vi "SUMMER SUNDAY BYTE[2].vi"() -> ()   [LabVIEW 2009]
uses:
  <vilib>/ULx/Create Channel.llb/ULx Create Channel (AI-Voltage-Basic).vi
  <vilib>/ULx/Read.llb/ULx Read (Analog DBL 1Chan 1Samp).vi
panel:
  out "POWER":bool
  out "data":dbl format="%_6g"
  out "xray":bool caption="BitValue"
  out "ENERGY LEVEL":dbl(knob) scale=0.0..15.0
  out "x*y":dbl
  out "Beam Pot":dbl format="%_6g"
  out "READY 2":bool
  out "DUMP":bool
  out "POWER":bool
  out "?":bool
  out "?":bool
  out "?":bool
  out "?":bool
  out "?":bool
  out "?":bool
  out "?":bool
  out "?":bool
  out "?":bool
  out "?":bool
  out "OPEN":bool
  out "CLOSED":bool
  out "READY":bool
  out "FAULT":bool
  out "MAGNET FORCE":dbl(slide) scale=0.0..10.0
  out "READY":bool
  out "TEMPERATURE":dbl(slide) scale=0.0..100.0
  in  "stop":bool
  out "?":bool
  out "?":bool
  out "?":bool
  out "?":bool
  out "FAULT":bool
  out "POWER":bool
  out "FLOW IN GPM":dbl(knob) scale=0.0..15.0
  # "USERS LAB AREA"
  # "BEAM STATUS"
  # "ROOM"
  # "XRAY"
  # "PUMP STATION"
  # "MAGNET STATUS"
  # "ORBIT"
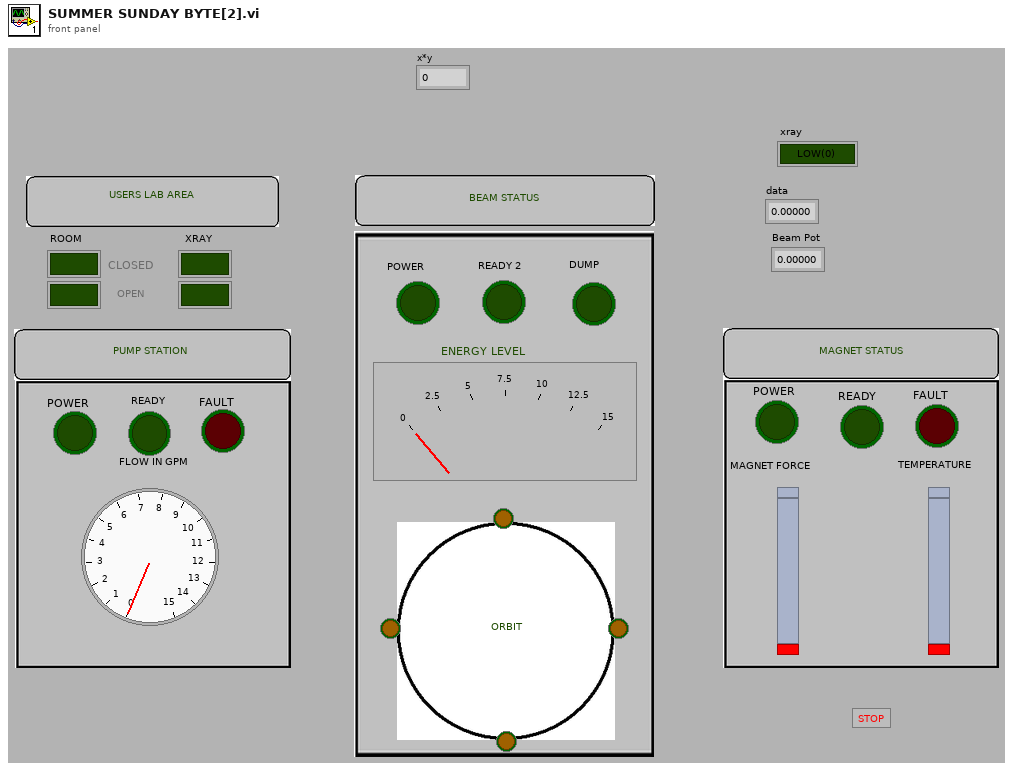
[diagram p1: front panel]
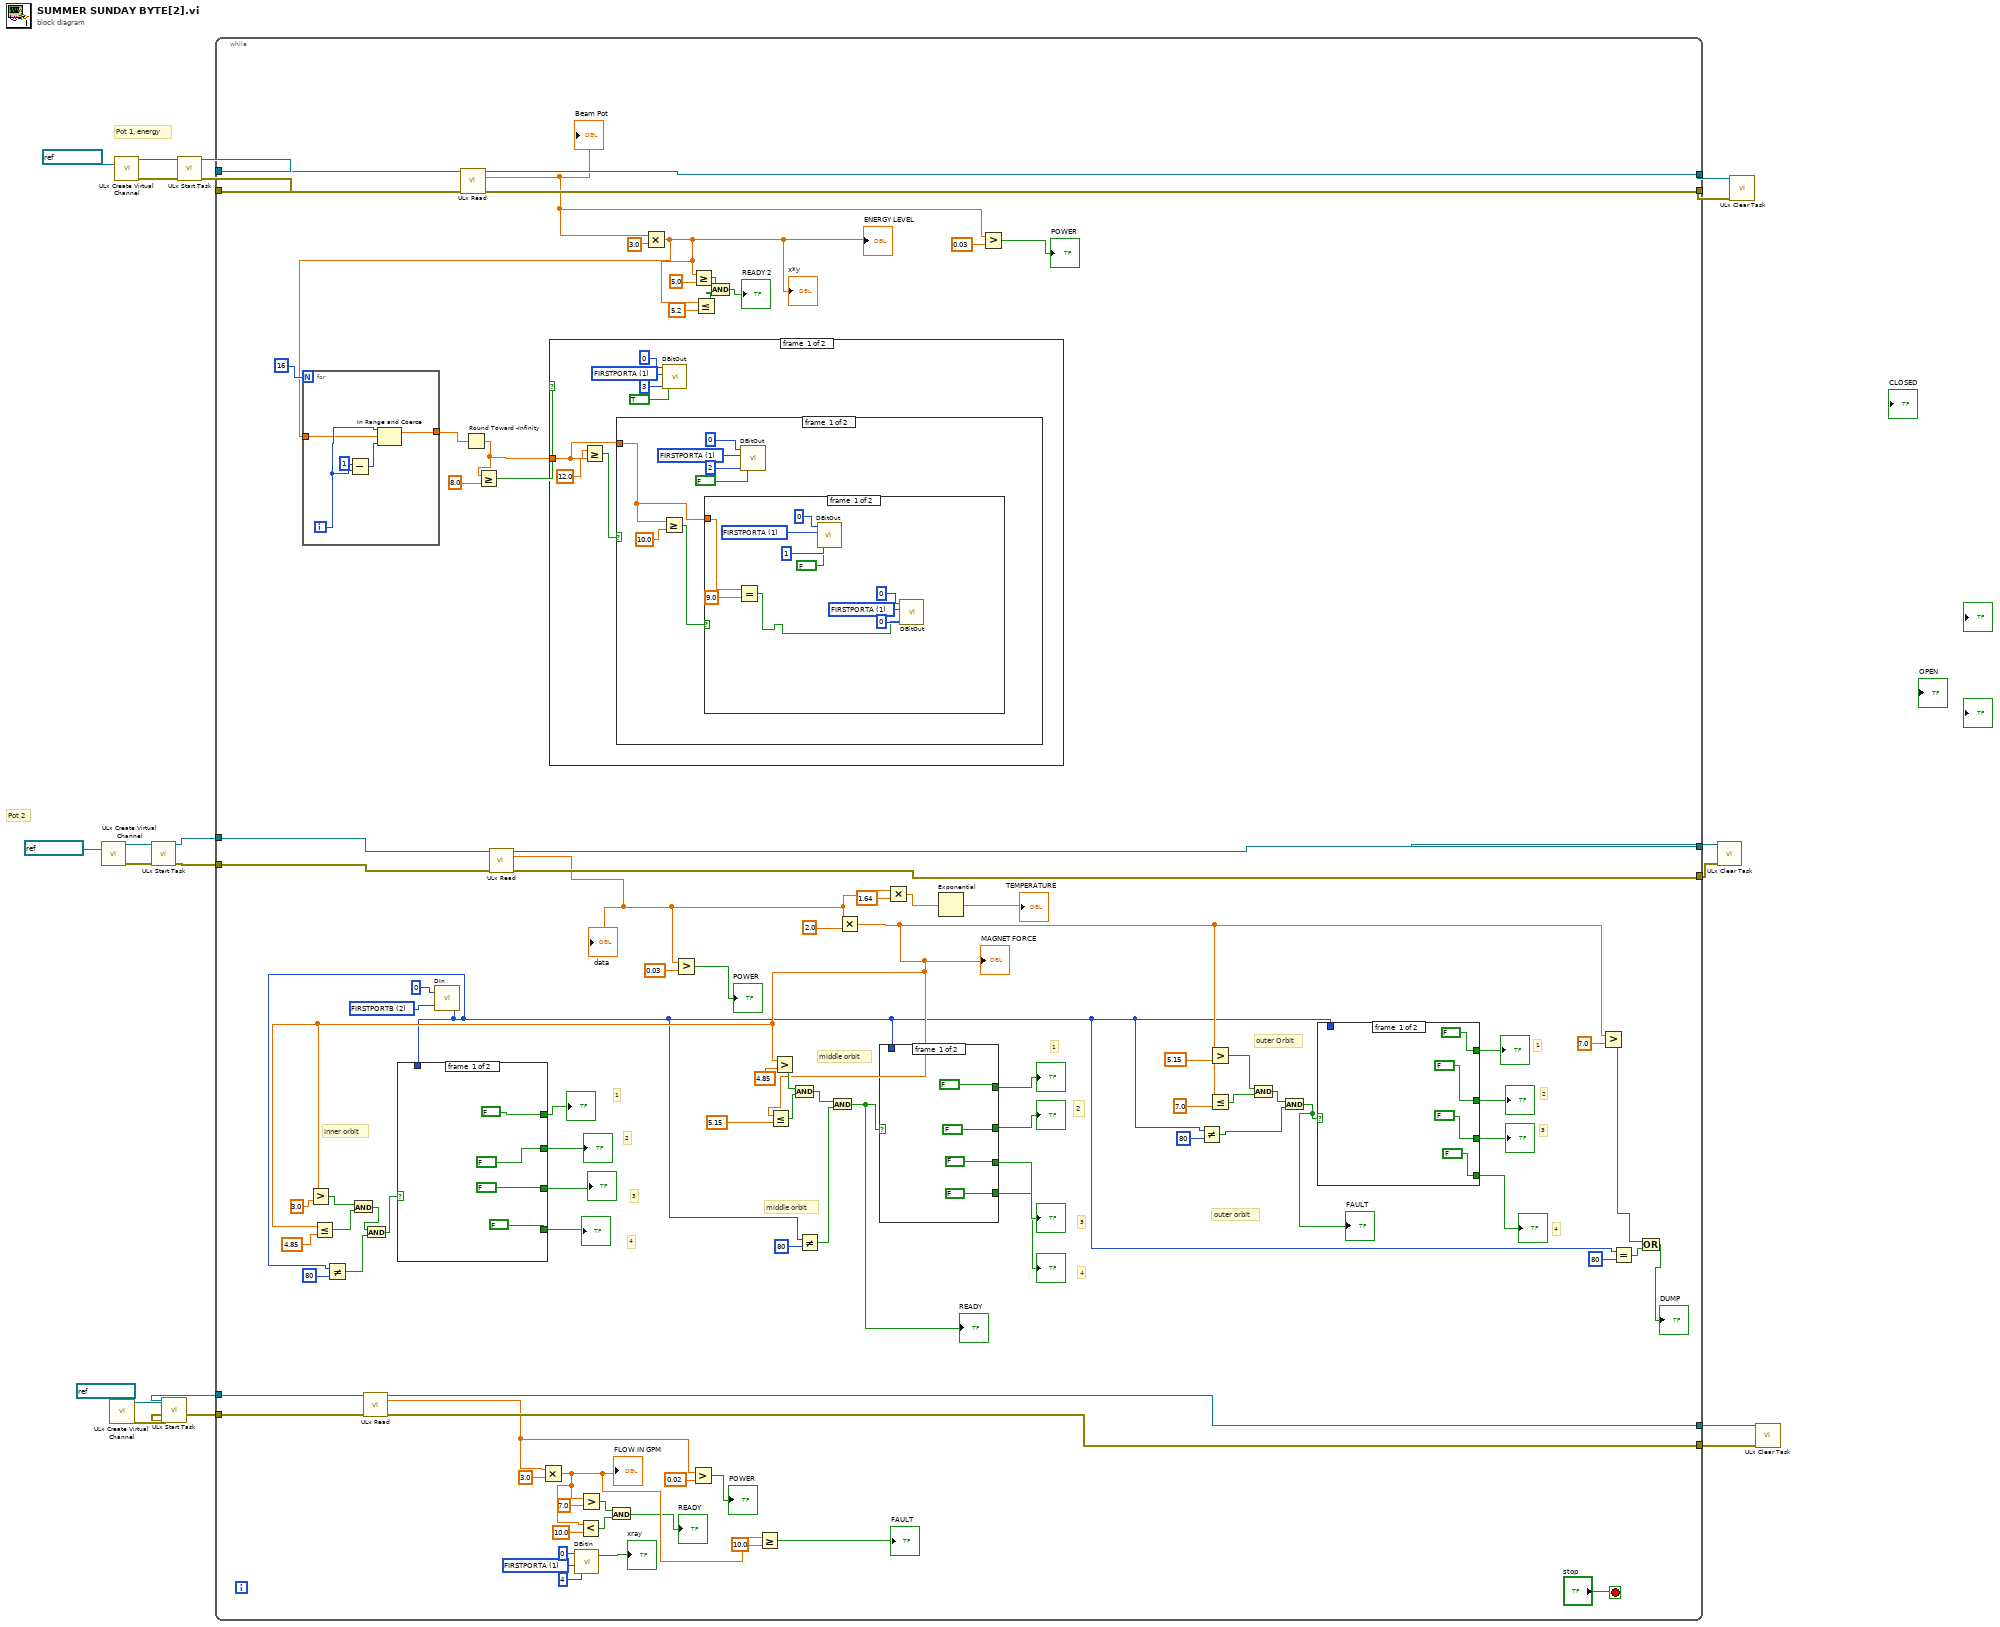
[diagram p0: block diagram]
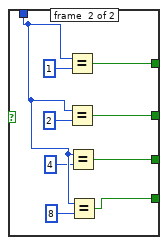
[diagram p2: hidden frame]
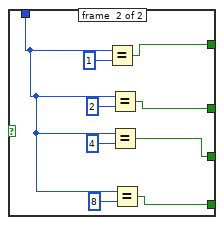
[diagram p3: hidden frame]
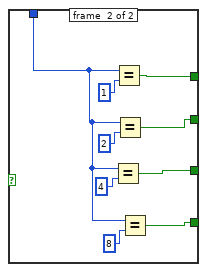
[diagram p4: hidden frame]
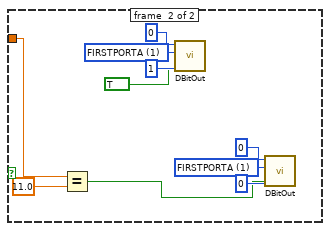
[diagram p5: hidden frame]
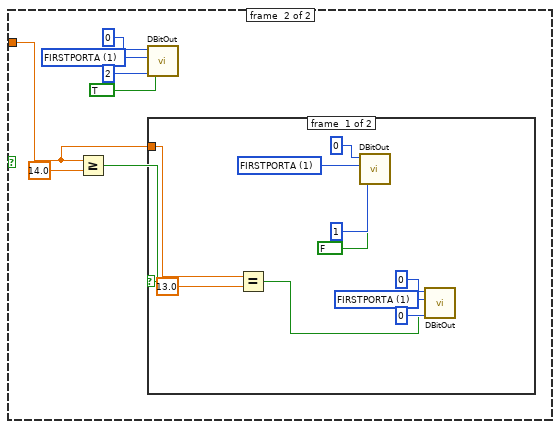
[diagram p6: hidden frame]
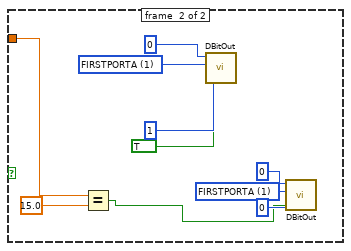
[diagram p7: hidden frame]
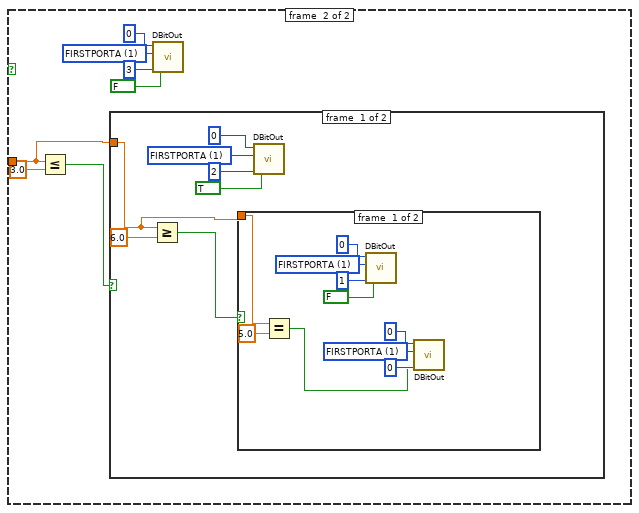
[diagram p8: hidden frame]
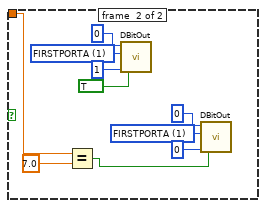
[diagram p9: hidden frame]
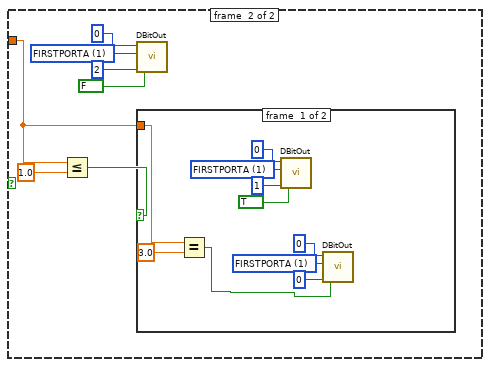
[diagram p10: hidden frame]
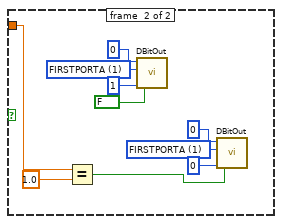
[diagram p11: hidden frame]
diagram:
  # "Pot 2"
  # "Pot 1, energy"
  n1 = call-poly <vilib>:"ULx Create Virtual Channel.vi"("physical channels"=refnum<k21> "Dev0/Ai1") -> ("task out"=w15:refnum<k24>, "error out"=w14:errorcluster)  [unwired: 13 in]
  n2 = call-poly <vilib>:"ULx Create Virtual Channel.vi"("physical channels"=refnum<k21> "Dev0/Ai2") -> ("task out"=w7:refnum<k24>, "error out"=w6:errorcluster)  [unwired: 13 in]
  n3 = call-poly <vilib>:"ULx Create Virtual Channel.vi"("physical channels"=refnum<k21> "Dev0/Ai0") -> ("task out"=w21:refnum<k24>, "error out"=w20:errorcluster)  [unwired: 13 in]
  n4 = call <vilib>:"ULx Start Task.vi"("task in"=w15, "error in"=w14) -> ("task out"=w13:refnum<k24>, "error out"=w12:errorcluster)  [unwired: 12 in]
  n5 = call <vilib>:"ULx Start Task.vi"("task in"=w7, "error in"=w6) -> ("task out"=w5:refnum<k24>, "error out"=w4:errorcluster)  [unwired: 12 in]
  n6 = call <vilib>:"ULx Start Task.vi"("task in"=w21, "error in"=w20) -> ("task out"=w19:refnum<k24>, "error out"=w18:errorcluster)  [unwired: 12 in]
  n7 = while {
    tunnel: w19 -> [w116]
    tunnel: w18 -> [w115]
    tunnel: [w114] -> w17
    tunnel: [w113] -> w16
    tunnel: w13 -> [w106]
    tunnel: w12 -> [w105]
    tunnel: [w104] -> w11
    tunnel: [w103] -> w10
    tunnel: w5 -> [w61]
    tunnel: w4 -> [w60]
    tunnel: [w59] -> w2
    tunnel: [w58] -> w1
    stop <- "stop" stop-if-true
    w56 = 1 items=["AUXPORT", "FIRSTPORTA"] ("PortType")
    w80 = 2 items=["AUXPORT", "FIRSTPORTA", "FIRSTPORTB", "FIRSTPORTCL", "FIRSTPORTCH", "SECONDPORTA", "SECONDPORTB", "SECONDPORTCL", "SECONDPORTCH", "THIRDPORTA", "THIRDPORTB", "THIRDPORTCL", "THIRDPORTCH", "FOURTHPORTA", "FOURTHPORTB", "FOURTHPORTCL", "FOURTHPORTCH", "FIFTHPORTA", "FIFTHPORTB", "FIFTHPORTCL", "FIFTHPORTCH", "SIXTHPORTA", "SIXTHPORTB", "SIXTHPORTCL", "SIXTHPORTCH", "SEVENTHPORTA", "SEVENTHPORTB", "SEVENTHPORTCL", "SEVENTHPORTCH", "EIGTHPORTA", "EIGHTHPORTB", "EIGHTHPORTCL", "EIGHTHPORTCH"] ("PortNum")
    # "outer Orbit"
    # "middle orbit"
    # "4"
    # "3"
    # "2"
    # "1"
    # "1"
    # "2"
    # "3"
    # "4"
    # "4"
    # "3"
    # "2"
    # "1"
    # "outer orbit"
    # "inner orbit"
    # "middle orbit"
    n8 = call-poly <vilib>:"ULx Read.vi"("task in"=w61, "error in"=w60) -> ("task out"=w59:refnum<k24>, "data"=w47:dbl, "error out"=w58:errorcluster)  [unwired: 11 in]
    n9 = call <menus>:"DIn.VI"("PortNum"=w80, "BoardNum"=u32 0) -> ("DataValue"=w68:i16)  [unwired: 1 out]
    n10 = Not Equal?(x=w68, y=i16 80) -> (x != y?=w90:bool)
    n11 = call-poly <vilib>:"ULx Read.vi"("task in"=w116, "error in"=w115) -> ("task out"=w114:refnum<k24>, "data"=w49:dbl, "error out"=w113:errorcluster)  [unwired: 11 in]
    "Beam Pot" <- w49
    n12 = call-poly <vilib>:"ULx Read.vi"("task in"=w106, "error in"=w105) -> ("task out"=w104:refnum<k24>, "data"=w25:dbl, "error out"=w103:errorcluster)  [unwired: 11 in]
    "data" <- w25
    n13 = Multiply(x=w47, y=3.0) -> (x*y=w32:dbl)
    "FLOW IN GPM" <- w32
    n14 = call <menus>:"DBitIn.VI"("BitNum"=4, "PortType"=w56, "BoardNum"=u32 0) -> ("BitValue"=→"xray":bool)  [unwired: 1 out]
    n15 = Less?(x=w32, y=10.0) -> (x < y?=w30:bool)
    n16 = Greater?(x=w32, y=7.0) -> (0:w31:bool)
    n17 = And(x=w31, y=w30) -> (x .and. y?=→"READY":bool)
    n18 = Multiply(x=w49, y=3.0) -> (x*y=w42:dbl)
    "x*y" <- w42
    "ENERGY LEVEL" <- w42
    n19 = for {
      N: 16 -> [_]
      tunnel: w42 -> [w280]
      tunnel: [w279] -> w110
      i -> [w282]
      n20 = Subtract(x=1, y=w282) -> (x-y=w283:i32)
      n21 = In Range and Coerce(upper limit=w282, x=w280, lower limit=w283) -> (coerced(x)=w279:dbl)  [unwired: 1 out]
    }
    n22 = Round Toward -Infinity(1:w110) -> (0:w107:dbl)
    n23 = Greater Or Equal?(x=w107, y=8.0) -> (x >= y?=w108:bool)
    n24 = case shown="False" w108 {
      tunnel: w107 -> [w157 w218]
      frame #0 {
        w162 = u32 1 items=["AUXPORT", "FIRSTPORTA"] ("PortType")
        n25 = Greater Or Equal?(x=w157, y=12.0) -> (x >= y?=w158:bool)
        n26 = case shown="True" w158 {
          tunnel: w157 -> [w164 w191]
          frame #0 {
            w169 = u32 1 items=["AUXPORT", "FIRSTPORTA"] ("PortType")
            n27 = Greater Or Equal?(x=w164, y=10.0) -> (x >= y?=w165:bool)
            n28 = case shown="True" w165 {
              tunnel: w164 -> [w176 w187]
              frame #0 {
                w174 = u32 1 items=["AUXPORT", "FIRSTPORTA"] ("PortType")
                w179 = u32 1 items=["AUXPORT", "FIRSTPORTA"] ("PortType")
                n29 = Equal?(x=w176, y=9.0) -> (x = y?=w171:bool)
                n30 = call <menus>:"DBitOut.VI"("BitValue"=FALSE, "BitNum"=u32 1, "PortType"=w179, "BoardNum"=u32 0) -> ()  [unwired: 1 out]
                n31 = call <menus>:"DBitOut.VI"("BitValue"=w171, "BitNum"=u32 0, "PortType"=w174, "BoardNum"=u32 0) -> ()  [unwired: 1 out]
              }
              frame #1 {
                w184 = u32 1 items=["AUXPORT", "FIRSTPORTA"] ("PortType")
                w189 = u32 1 items=["AUXPORT", "FIRSTPORTA"] ("PortType")
                n32 = Equal?(x=w187, y=11.0) -> (x = y?=w181:bool)
                n33 = call <menus>:"DBitOut.VI"("BitValue"=TRUE, "BitNum"=u32 1, "PortType"=w189, "BoardNum"=u32 0) -> ()  [unwired: 1 out]
                n34 = call <menus>:"DBitOut.VI"("BitValue"=w181, "BitNum"=u32 0, "PortType"=w184, "BoardNum"=u32 0) -> ()  [unwired: 1 out]
              }
            }
            n35 = call <menus>:"DBitOut.VI"("BitValue"=FALSE, "BitNum"=u32 2, "PortType"=w169, "BoardNum"=u32 0) -> ()  [unwired: 1 out]
          }
          frame #1 {
            w196 = u32 1 items=["AUXPORT", "FIRSTPORTA"] ("PortType")
            n36 = Greater Or Equal?(x=w191, y=14.0) -> (x >= y?=w192:bool)
            n37 = call <menus>:"DBitOut.VI"("BitValue"=TRUE, "BitNum"=u32 2, "PortType"=w196, "BoardNum"=u32 0) -> ()  [unwired: 1 out]
            n38 = case shown="False" w192 {
              tunnel: w191 -> [w203 w213]
              frame #0 {
                w201 = u32 1 items=["AUXPORT", "FIRSTPORTA"] ("PortType")
                w206 = u32 1 items=["AUXPORT", "FIRSTPORTA"] ("PortType")
                n39 = Equal?(x=w203, y=13.0) -> (x = y?=w198:bool)
                n40 = call <menus>:"DBitOut.VI"("BitValue"=FALSE, "BitNum"=u32 1, "PortType"=w206, "BoardNum"=u32 0) -> ()  [unwired: 1 out]
                n41 = call <menus>:"DBitOut.VI"("BitValue"=w198, "BitNum"=u32 0, "PortType"=w201, "BoardNum"=u32 0) -> ()  [unwired: 1 out]
              }
              frame #1 {
                w211 = u32 1 items=["AUXPORT", "FIRSTPORTA"] ("PortType")
                w216 = u32 1 items=["AUXPORT", "FIRSTPORTA"] ("PortType")
                n42 = Equal?(x=w213, y=15.0) -> (x = y?=w208:bool)
                n43 = call <menus>:"DBitOut.VI"("BitValue"=TRUE, "BitNum"=u32 1, "PortType"=w216, "BoardNum"=u32 0) -> ()  [unwired: 1 out]
                n44 = call <menus>:"DBitOut.VI"("BitValue"=w208, "BitNum"=u32 0, "PortType"=w211, "BoardNum"=u32 0) -> ()  [unwired: 1 out]
              }
            }
          }
        }
        n45 = call <menus>:"DBitOut.VI"("BitValue"=TRUE, "BitNum"=u32 3, "PortType"=w162, "BoardNum"=u32 0) -> ()  [unwired: 1 out]
      }
      frame #1 {
        w223 = u32 1 items=["AUXPORT", "FIRSTPORTA"] ("PortType")
        n46 = Less Or Equal?(x=w218, y=3.0) -> (x <= y?=w219:bool)
        n47 = case shown="False" w219 {
          tunnel: w218 -> [w225 w252]
          frame #0 {
            w230 = u32 1 items=["AUXPORT", "FIRSTPORTA"] ("PortType")
            n48 = Greater Or Equal?(x=w225, y=6.0) -> (x >= y?=w226:bool)
            n49 = case shown="False" w226 {
              tunnel: w225 -> [w234 w247]
              frame #0 {
                w236 = u32 1 items=["AUXPORT", "FIRSTPORTA"] ("PortType")
                w240 = u32 1 items=["AUXPORT", "FIRSTPORTA"] ("PortType")
                n50 = Equal?(x=w234, y=5.0) -> (x = y?=w232:bool)
                n51 = call <menus>:"DBitOut.VI"("BitValue"=FALSE, "BitNum"=u32 1, "PortType"=w240, "BoardNum"=u32 0) -> ()  [unwired: 1 out]
                n52 = call <menus>:"DBitOut.VI"("BitValue"=w232, "BitNum"=u32 0, "PortType"=w236, "BoardNum"=u32 0) -> ()  [unwired: 1 out]
              }
              frame #1 {
                w244 = u32 1 items=["AUXPORT", "FIRSTPORTA"] ("PortType")
                w250 = u32 1 items=["AUXPORT", "FIRSTPORTA"] ("PortType")
                n53 = Equal?(x=w247, y=7.0) -> (x = y?=w242:bool)
                n54 = call <menus>:"DBitOut.VI"("BitValue"=TRUE, "BitNum"=u32 1, "PortType"=w250, "BoardNum"=u32 0) -> ()  [unwired: 1 out]
                n55 = call <menus>:"DBitOut.VI"("BitValue"=w242, "BitNum"=u32 0, "PortType"=w244, "BoardNum"=u32 0) -> ()  [unwired: 1 out]
              }
            }
            n56 = call <menus>:"DBitOut.VI"("BitValue"=TRUE, "BitNum"=u32 2, "PortType"=w230, "BoardNum"=u32 0) -> ()  [unwired: 1 out]
          }
          frame #1 {
            w257 = u32 1 items=["AUXPORT", "FIRSTPORTA"] ("PortType")
            n57 = Less Or Equal?(x=w252, y=1.0) -> (x <= y?=w253:bool)
            n58 = call <menus>:"DBitOut.VI"("BitValue"=FALSE, "BitNum"=u32 2, "PortType"=w257, "BoardNum"=u32 0) -> ()  [unwired: 1 out]
            n59 = case shown="True" w253 {
              tunnel: w252 -> [w264 w274]
              frame #0 {
                w261 = u32 1 items=["AUXPORT", "FIRSTPORTA"] ("PortType")
                w267 = u32 1 items=["AUXPORT", "FIRSTPORTA"] ("PortType")
                n60 = Equal?(x=w264, y=3.0) -> (x = y?=w259:bool)
                n61 = call <menus>:"DBitOut.VI"("BitValue"=TRUE, "BitNum"=u32 1, "PortType"=w267, "BoardNum"=u32 0) -> ()  [unwired: 1 out]
                n62 = call <menus>:"DBitOut.VI"("BitValue"=w259, "BitNum"=u32 0, "PortType"=w261, "BoardNum"=u32 0) -> ()  [unwired: 1 out]
              }
              frame #1 {
                w271 = u32 1 items=["AUXPORT", "FIRSTPORTA"] ("PortType")
                w277 = u32 1 items=["AUXPORT", "FIRSTPORTA"] ("PortType")
                n63 = Equal?(x=w274, y=1.0) -> (x = y?=w269:bool)
                n64 = call <menus>:"DBitOut.VI"("BitValue"=FALSE, "BitNum"=u32 1, "PortType"=w277, "BoardNum"=u32 0) -> ()  [unwired: 1 out]
                n65 = call <menus>:"DBitOut.VI"("BitValue"=w269, "BitNum"=u32 0, "PortType"=w271, "BoardNum"=u32 0) -> ()  [unwired: 1 out]
              }
            }
          }
        }
        n66 = call <menus>:"DBitOut.VI"("BitValue"=FALSE, "BitNum"=u32 3, "PortType"=w223, "BoardNum"=u32 0) -> ()  [unwired: 1 out]
      }
    }
    n67 = Greater?(x=w25, y=0.03) -> (0:→"POWER":bool)
    n68 = Greater?(x=w47, y=0.02) -> (0:→"POWER":bool)
    n69 = Greater Or Equal?(x=w42, y=5.0) -> (x >= y?=w39:bool)
    n70 = Less Or Equal?(x=w42, y=5.2) -> (x <= y?=w38:bool)
    n71 = And(x=w39, y=w38) -> (x .and. y?=→"READY 2":bool)
    n72 = Greater Or Equal?(x=w32, y=10.0) -> (x >= y?=→"FAULT":bool)
    n73 = Not Equal?(x=w68, y=i16 80) -> (x != y?=w76:bool)
    n74 = Multiply(x=w25, y=2.0) -> (x*y=w83:dbl)
    "MAGNET FORCE" <- w83
    n75 = Greater?(x=w83, y=3.0) -> (0:w99:bool)
    n76 = Less Or Equal?(x=w83, y=4.85) -> (x <= y?=w100:bool)
    n77 = And(x=w99, y=w100) -> (x .and. y?=w92:bool)
    n78 = And(x=w92, y=w90) -> (x .and. y?=w91:bool)
    n79 = case shown="True" w91 {
      tunnel: [FALSE w151] -> w64
      tunnel: [FALSE w150] -> w65
      tunnel: [FALSE w149] -> w62
      tunnel: [FALSE w148] -> w63
      tunnel: w68 -> [_ w156]
      frame #0 {
      }
      frame #1 {
        n80 = Equal?(x=w156, y=i16 4) -> (x = y?=w149:bool)
        n81 = Equal?(x=w156, y=i16 1) -> (x = y?=w151:bool)
        n82 = Equal?(x=w156, y=i16 2) -> (x = y?=w150:bool)
        n83 = Equal?(x=w156, y=i16 8) -> (x = y?=w148:bool)
      }
    }
    "?" <- w65
    "?" <- w62
    "?" <- w63
    "?" <- w64
    n84 = Less Or Equal?(x=w83, y=5.15) -> (x <= y?=w96:bool)
    n85 = Greater?(x=w83, y=4.85) -> (0:w97:bool)
    n86 = And(x=w97, y=w96) -> (x .and. y?=w89:bool)
    n87 = And(x=w89, y=w76) -> (x .and. y?=w45:bool)
    "READY" <- w45
    n88 = case shown="True" w45 {
      tunnel: [FALSE w130] -> w75
      tunnel: [FALSE w129] -> w74
      tunnel: [FALSE w128] -> w73
      tunnel: [FALSE w127] -> w72
      tunnel: w68 -> [_ w126]
      frame #0 {
      }
      frame #1 {
        n89 = Equal?(x=w126, y=i16 1) -> (x = y?=w130:bool)
        n90 = Equal?(x=w126, y=i16 2) -> (x = y?=w129:bool)
        n91 = Equal?(x=w126, y=i16 4) -> (x = y?=w128:bool)
        n92 = Equal?(x=w126, y=i16 8) -> (x = y?=w127:bool)
      }
    }
    "?" <- w75
    "?" <- w74
    "?" <- w73
    "?" <- w72
    n93 = Multiply(x=w25, y=1.64) -> (x*y=w23:dbl)
    n94 = Exponential(1:w23) -> (0:→"TEMPERATURE":dbl)
    n95 = Greater?(x=w49, y=0.03) -> (0:→"POWER":bool)
    n96 = Not Equal?(x=w68, y=i16 80) -> (x != y?=w70:bool)
    n97 = Greater?(x=w83, y=5.15) -> (0:w94:bool)
    n98 = Less Or Equal?(x=w83, y=7.0) -> (x <= y?=w93:bool)
    n99 = And(x=w94, y=w93) -> (x .and. y?=w82:bool)
    n100 = And(x=w82, y=w70) -> (x .and. y?=w26:bool)
    "FAULT" <- w26
    n101 = case shown="True" w26 {
      tunnel: [FALSE w135] -> w87
      tunnel: [FALSE w136] -> w86
      tunnel: [FALSE w137] -> w85
      tunnel: [FALSE w138] -> w84
      tunnel: w68 -> [_ w143]
      frame #0 {
      }
      frame #1 {
        n102 = Equal?(x=w143, y=i16 1) -> (x = y?=w138:bool)
        n103 = Equal?(x=w143, y=i16 2) -> (x = y?=w137:bool)
        n104 = Equal?(x=w143, y=i16 4) -> (x = y?=w136:bool)
        n105 = Equal?(x=w143, y=i16 8) -> (x = y?=w135:bool)
      }
    }
    "?" <- w84
    "?" <- w85
    "?" <- w86
    "?" <- w87
    n106 = Greater?(x=w83, y=7.0) -> (0:w27:bool)
    n107 = Equal?(x=w68, y=i16 80) -> (x = y?=w66:bool)
    n108 = Or(x=w27, y=w66) -> (x .or. y?=→"DUMP":bool)
  }
  n109 = call <vilib>:"ULx Clear Task.vi"("task in"=w11, "error in"=w10) -> ()  [unwired: 13 in, 1 out]
  n110 = call <vilib>:"ULx Clear Task.vi"("task in"=w17, "error in"=w16) -> ()  [unwired: 13 in, 1 out]
  n111 = call <vilib>:"ULx Clear Task.vi"("task in"=w2, "error in"=w1) -> ()  [unwired: 13 in, 1 out]
